vi "Configure Runt Trigger Source.vi"(0 "VISA Resource Name":refnum<visa-resource-name>, 1 "Runt Polarity (Positive)":i32(slide), 5 "Trigger Source (Channel 1)":string(combo)="CH1", 7 "Runt Low Threshold (1.0 V)":dbl=1.0 format="%.2p", 9 "Runt High Threshold (4.0 V)":dbl=4.0 format="%.2p", 11 "error in (no error)":errorcluster {"code" format="%.0x"}) -> (4 "VISA Resource Name Out":refnum<visa-resource-name>, 15 "error out":errorcluster {"code" format="%.0x"})   [LabVIEW 2010, in "Tektronix TDS 3000 Series.lvlib"]
doc: "This VI configures the runt trigger. A runt trigger occurs when the trigger signal crosses one of the runt thresholds twice without crossing the other runt threshold. You specify the runt thresholds with the Runt Low Threshold and Runt High Threshold controls. You specify the polarity of the runt with the Runt Polarity control.\n\nNotes:\n\n(1) This VI affects instrument behavior only if the Trigger Type is Runt Trigger. Call the Configure Trigger VI to set the Trigger Type before you call this VI."
uses:
  <instrlib>/Tektronix TDS 3000 Series/Tektronix TDS 3000 Series.lvlib
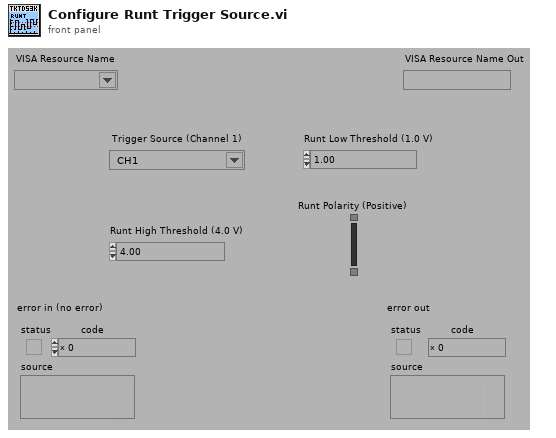
[diagram p1: front panel]
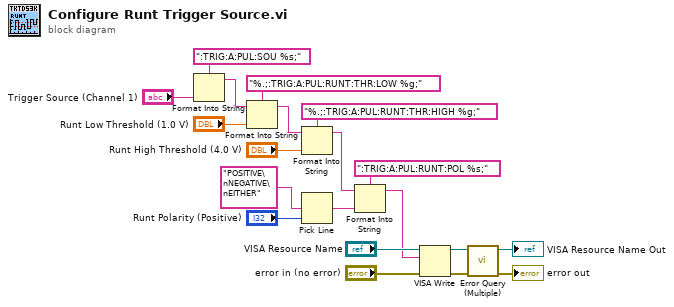
[diagram p0: block diagram]
diagram:
  n1 = Format Into String(format string=":TRIG:A:PUL:SOU %s;", "Trigger Source (Channel 1)") -> (resulting string=w8:string)  [unwired: 2 in, 1 out]
  n2 = Format Into String(format string="%.;:TRIG:A:PUL:RUNT:THR:LOW %g;", initial string=w8, "Runt Low Threshold (1.0 V)") -> (resulting string=w6:string)  [unwired: 1 in, 1 out]
  n3 = Format Into String(format string="%.;:TRIG:A:PUL:RUNT:THR:HIGH %g;", initial string=w6, "Runt High Threshold (4.0 V)") -> (resulting string=w9:string)  [unwired: 1 in, 1 out]
  n4 = Pick Line(multi-line string="POSITIVE\nNEGATIVE\nEITHER", line index="Runt Polarity (Positive)") -> (output string=w11:string)  [unwired: 1 in]
  n5 = Format Into String(format string=":TRIG:A:PUL:RUNT:POL %s;", initial string=w9, w11) -> (resulting string=w5:string)  [unwired: 1 in, 1 out]
  n6 = VISA Write(VISA resource name="VISA Resource Name", write buffer=w5, error in (no error)="error in (no error)") -> (VISA resource name out=w4:refnum<visa-resource-name>, error out=w3:errorcluster)  [unwired: 1 out]
  n7 = call <instrlib>:"Error Query (Multiple).vi"("error in (no error)"=w3, "VISA Resource Name"=w4) -> ("error out"=→"error out":errorcluster, "VISA Resource Name Out"=→"VISA Resource Name Out":refnum<visa-resource-name>)  [unwired: 6 in, 2 out]
